vi "NextState.vi"(0 "object in":refnum<class "InterceptBallTactic.lvclass">, 4 "GameRef":refnum<data-value>, 5 "error in (no error)":errorcluster) -> (14 "object out":refnum<class "InterceptBallTactic.lvclass">, 19 "error out":errorcluster)   [LabVIEW 2023, in "InterceptBallTactic.lvclass"]
uses:
  InterceptBallTactic.lvclass
  Zone_class/Zone.lvclass
  Robot_class/Robot.lvclass
  Utilities_class/Utilities.lvclass
  Game_class/Game.lvclass
panel:
  in  "Robot in":refnum<class "Robot.lvclass">
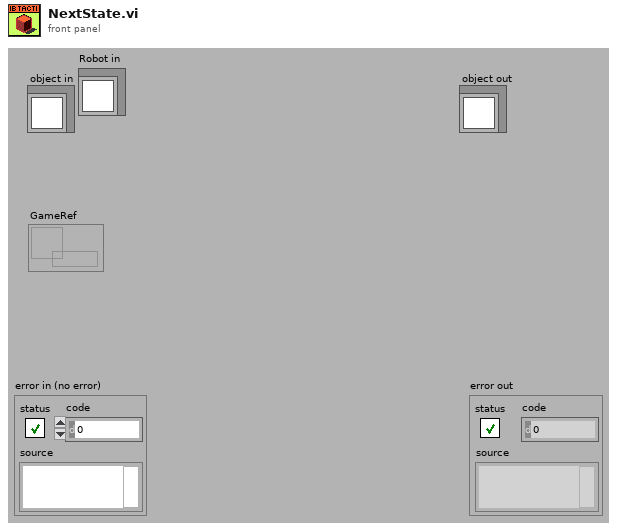
[diagram p1: front panel]
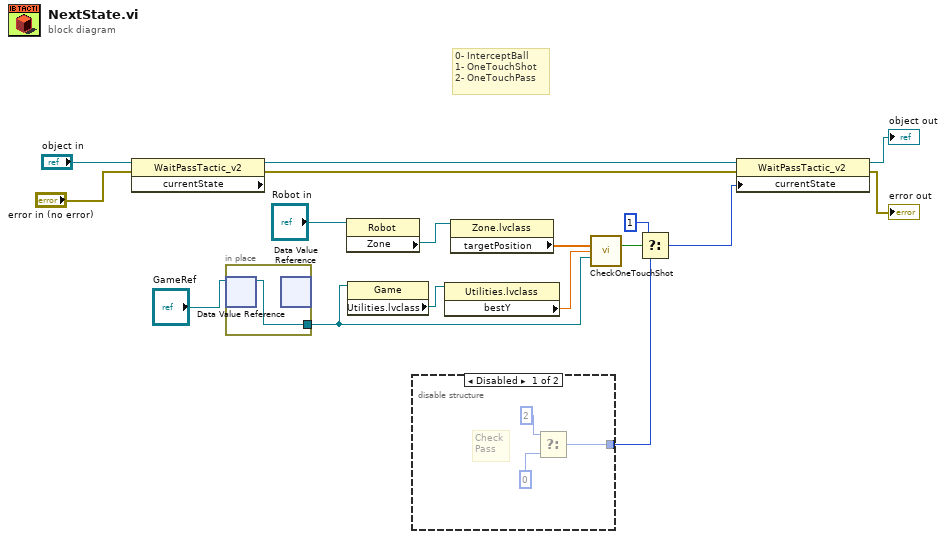
[diagram p0: block diagram]
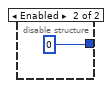
[diagram p2: hidden frame]
diagram:
  # "0- InterceptBall\n1- OneTouchShot\n2- OneTouchPass"
  n1 = property class="WaitPassTactic_v2" props=["currentState"](reference="object in", error in="error in (no error)") -> (reference out=w17:refnum<class "InterceptBallTactic.lvclass">, error out=w16:errorcluster)  [unwired: 1 out]
  n2 = in-place {
    in-place-border: [w18] -> w9
    n3 = in-place-dvr #1("GameRef") -> (w18:refnum<class "Game.lvclass">)  [unwired: 1 out]
    n4 = in-place-dvr #1() -> ()  [unwired: 1 in, 2 out]
  }
  n5 = property class="Robot"(reference="Robot in") -> ("Zone"=w5:refnum<class "Zone.lvclass">)  [unwired: 1 in, 2 out]
  n6 = property class="Game"(reference=w9) -> ("Utilities.lvclass"=w8:refnum<class "Utilities.lvclass">)  [unwired: 1 in, 2 out]
  n7 = disable-structure shown="Disabled" {
    disable-tunnel: [w21 0] -> w11
    frame Disabled {
      # "Check\nPass"
      n8 = Select(t=2, f=0) -> (s? t:f=w21:i32)  [unwired: 1 in]
    }
    frame Enabled {
    }
  }
  n9 = property class="Utilities.lvclass"(reference=w8) -> ("bestY"=w7:dbl)  [unwired: 1 in, 2 out]
  n10 = property class="Zone.lvclass"(reference=w5) -> ("targetPosition"=w4:dbl[])  [unwired: 1 in, 2 out]
  n11 = call-dynamic "CheckOneTouchShot.vi"("Point"=w4, "Best y"=w7, "Game"=w9) -> ("OneTouch"=w1:bool)  [unwired: 9 in, 3 out]
  n12 = Select(t=1, s=w1, f=w11) -> (s? t:f=w10:i32)
  n13 = property class="WaitPassTactic_v2"(reference=w17, error in=w16, "currentState"=w10) -> (reference out=→"object out":refnum<class "InterceptBallTactic.lvclass">, error out=→"error out":errorcluster)
